vi "GlobalSetGetConfigureCamera.vi"() -> ()   [LabVIEW 2013]
panel:
  in  "Kinetics":sgl
  in  "gain":i32
  in  "Hbin":i32
  in  "Exposure":sgl
  in  "Vbin":i32
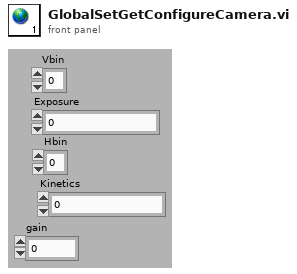
[diagram p1: front panel]
diagram:
